vi "GeoData.vi"() -> ()   [LabVIEW 2017] (continued)
Pence springs\tWV\tSummers County\tH1\n24943\t54089\tGrassy meadows\tWV\tSummers County\tH1\n26330\t54091\tBridgeport\tWV\tTaylor County\tH1\n26374\t54091\tIndependence\tWV\tTaylor County\tH1\n26416\t54091\tPhilippi\tWV\tTaylor County\tH1\n26435\t54091\tSimpson\tWV\tTaylor County\tH1\n26354\t54091\tGrafton\tWV\tTaylor County\tH1\n26347\t54091\tFlemington\tWV\tTaylor County\tH1\n26554\t54091\tFairmont\tWV\tTaylor County\tH1\n26440\t54091\tThornton\tWV\tTaylor County\tH1\n26431\t54091\tShinnston\tWV\tTaylor County\tH1\n26424\t54091\tRosemont\tWV\tTaylor County\tH1\n26287\t54093\tParsons\tWV\tTucker County\tH1\n26271\t54093\tHendricks\tWV\tTucker County\tH1\n26263\t54093\tDryfork\tWV\tTucker County\tH1\n26254\t54093\tBowden\tWV\tTucker County\tH1\n26260\t54093\tDavis\tWV\tTucker County\tH1\n26289\t54093\tRed creek\tWV\tTucker County\tH1\n26283\t54093\tMontrose\tWV\tTucker County\tH1\n26276\t54093\tKerens\tWV\tTucker County\tH1\n26269\t54093\tHambleton\tWV\tTucker County\tH1\n26270\t54093\tHarman\tWV\tTucker County\tH1\n26292\t54093\tThomas\tWV\tTucker County\tH1\n26170\t54095\tSaint marys\tWV\tTyler County\tH1\n26415\t54095\tPennsboro\tWV\tTyler County\tH1\n26456\t54095\tWest union\tWV\tTyler County\tH1\n26155\t54095\tNew martinsville\tWV\tTyler County\tH1\n26159\t54095\tPaden city\tWV\tTyler County\tH1\n26175\t54095\tSistersville\tWV\tTyler County\tH1\n26149\t54095\tMiddlebourne\tWV\tTyler County\tH1\n26320\t54095\tAlma\tWV\tTyler County\tH1\n26167\t54095\tReader\tWV\tTyler County\tH1\n26377\t54095\tJacksonburg\tWV\tTyler County\tH1\n26146\t54095\tFriendly\tWV\tTyler County\tH1\n26434\t54095\tShirley\tWV\tTyler County\tH1\n26267\t54097\tEllamore\tWV\tUpshur County\tH1\n26218\t54097\tFrench creek\tWV\tUpshur County\tH1\n26385\t54097\tLost creek\tWV\tUpshur County\tH1\n26372\t54097\tHorner\tWV\tUpshur County\tH1\n26215\t54097\tCleveland\tWV\tUpshur County\tH1\n26236\t54097\tSelbyville\tWV\tUpshur County\tH1\n26210\t54097\tAdrian\tWV\tUpshur County\tH1\n26201\t54097\tBuckhannon\tWV\tUpshur County\tH1\n26343\t54097\tCrawford\tWV\tUpshur County\tH1\n26228\t54097\tKanawha head\tWV\tUpshur County\tH1\n26229\t54097\tLorentz\tWV\tUpshur County\tH1\n26234\t54097\tRock cave\tWV\tUpshur County\tH1\n26238\t54097\tVolga\tWV\tUpshur County\tH1\n26237\t54097\tTallmansville\tWV\tUpshur County\tH1\n25504\t54099\tBarboursville\tWV\tWayne County\tH1\n25530\t54099\tKenova\tWV\tWayne County\tH1\n25701\t54099\tHuntington\tWV\tWayne County\tH1\n25704\t54099\tHuntington\tWV\tWayne County\tH1\n25514\t54099\tFort gay\tWV\tWayne County\tH1\n25517\t54099\tGenoa\tWV\tWayne County\tH1\n25555\t54099\tPrichard\tWV\tWayne County\tH1\n25699\t54099\tWilsondale\tWV\tWayne County\tH1\n25524\t54099\tHarts\tWV\tWayne County\tH1\n25511\t54099\tDunlow\tWV\tWayne County\tH1\n25669\t54099\tCrum\tWV\tWayne County\tH1\n25562\t54099\tShoals\tWV\tWayne County\tH1\n25671\t54099\tDingess\tWV\tWayne County\tH1\n25534\t54099\tKiahsville\tWV\tWayne County\tH1\n25512\t54099\tEast lynn\tWV\tWayne County\tH1\n25570\t54099\tWayne\tWV\tWayne County\tH1\n25535\t54099\tLavalette\tWV\tWayne County\tH1\n25557\t54099\tRanger\tWV\tWayne County\tH1\n25507\t54099\tCeredo\tWV\tWayne County\tH1\n25674\t54099\tKermit\tWV\tWayne County\tH1\n25506\t54099\tBranchland\tWV\tWayne County\tH1\n26217\t54101\tDiana\tWV\tWebster County\tH1\n26203\t54101\tErbacon\tWV\tWebster County\tH1\n26266\t54101\tUpperglade\tWV\tWebster County\tH1\n26288\t54101\tWebster springs\tWV\tWebster County\tH1\n26208\t54101\tCamden on gauley\tWV\tWebster County\tH1\n26610\t54101\tBirch river\tWV\tWebster County\tH1\n26222\t54101\tHacker valley\tWV\tWebster County\tH1\n26206\t54101\tCowen\tWV\tWebster County\tH1\n26298\t54101\tBergoo\tWV\tWebster County\tH1\n26033\t54103\tCameron\tWV\tWetzel County\tH1\n26562\t54103\tBurton\tWV\tWetzel County\tH1\n26582\t54103\tMannington\tWV\tWetzel County\tH1\n26581\t54103\tLittleton\tWV\tWetzel County\tH1\n26437\t54103\tSmithfield\tWV\tWetzel County\tH1\n26162\t54103\tPorters falls\tWV\tWetzel County\tH1\n26155\t54103\tNew martinsville\tWV\tWetzel County\tH1\n26585\t54103\tMetz\tWV\tWetzel County\tH1\n26159\t54103\tPaden city\tWV\tWetzel County\tH1\n26575\t54103\tHundred\tWV\tWetzel County\tH1\n26561\t54103\tBig run\tWV\tWetzel County\tH1\n26055\t54103\tProctor\tWV\tWetzel County\tH1\n26149\t54103\tMiddlebourne\tWV\tWetzel County\tH1\n26348\t54103\tFolsom\tWV\tWetzel County\tH1\n26167\t54103\tReader\tWV\tWetzel County\tH1\n26377\t54103\tJacksonburg\tWV\tWetzel County\tH1\n26419\t54103\tPine grove\tWV\tWetzel County\tH1\n25252\t54105\tLe roy\tWV\tWirt County\tH1\n26180\t54105\tWalker\tWV\tWirt County\tH1\n25275\t54105\tSandyville\tWV\tWirt County\tH1\n26161\t54105\tPetroleum\tWV\tWirt County\tH1\n26141\t54105\tCreston\tWV\tWirt County\tH1\n26143\t54105\tElizabeth\tWV\tWirt County\tH1\n26160\t54105\tPalestine\tWV\tWirt County\tH1\n26152\t54105\tMunday\tWV\tWirt County\tH1\n25270\t54105\tReedy\tWV\tWirt County\tH1\n26138\t54105\tBrohard\tWV\tWirt County\tH1\n26169\t54107\tRockport\tWV\tWood County\tH1\n26170\t54107\tSaint marys\tWV\tWood County\tH1\n26184\t54107\tWaverly\tWV\tWood County\tH1\n26180\t54107\tWalker\tWV\tWood County\tH1\n26102\t54107\tParkersburg\tWV\tWood County\tH1\n26101\t54107\tParkersburg\tWV\tWood County\tH1\n26164\t54107\tRavenswood\tWV\tWood County\tH1\n26142\t54107\tDavisville\tWV\tWood County\tH1\n26103\t54107\tParkersburg\tWV\tWood County\tH1\n26150\t54107\tMineral wells\tWV\tWood County\tH1\n26120\t54107\tMineral wells\tWV\tWood County\tH1\n26104\t54107\tParkersburg\tWV\tWood County\tH1\n26181\t54107\tWashington\tWV\tWood County\tH1\n26143\t54107\tElizabeth\tWV\tWood County\tH1\n26187\t54107\tWilliamstown\tWV\tWood County\tH1\n26106\t54107\tParkersburg\tWV\tWood County\tH1\n26133\t54107\tBelleville\tWV\tWood County\tH1\n26121\t54107\tMineral wells\tWV\tWood County\tH1\n26105\t54107\tVienna\tWV\tWood County\tH1\n24870\t54109\tOceana\tWV\tWyoming County\tH1\n25882\t54109\tMullens\tWV\tWyoming County\tH1\n25617\t54109\tDavin\tWV\tWyoming County\tH1\n24716\t54109\tBud\tWV\tWyoming County\tH1\n25875\t54109\tMc graws\tWV\tWyoming County\tH1\n24726\t54109\tHerndon\tWV\tWyoming County\tH1\n24827\t54109\tCyclone\tWV\tWyoming County\tH1\n25870\t54109\tMaben\tWV\tWyoming County\tH1\n24898\t54109\tWyoming\tWV\tWyoming County\tH1\n25943\t54109\tWyco\tWV\tWyoming County\tH1\n24828\t54109\tDavy\tWV\tWyoming County\tH1\n25928\t54109\tStephenson\tWV\tWyoming County\tH1\n25826\t54109\tCorinne\tWV\tWyoming County\tH1\n25810\t54109\tAllen junction\tWV\tWyoming County\tH1\n24857\t54109\tLynco\tWV\tWyoming County\tH1\n25876\t54109\tSaulsville\tWV\tWyoming County\tH1\n24882\t54109\tSimon\tWV\tWyoming County\tH1\n25913\t54109\tRavencliff\tWV\tWyoming County\tH1\n24854\t54109\tKopperston\tWV\tWyoming County\tH1\n24736\t54109\tMatoaka\tWV\tWyoming County\tH1\n24839\t54109\tHanover\tWV\tWyoming County\tH1\n24849\t54109\tJesse\tWV\tWyoming County\tH1\n25848\t54109\tGlen rogers\tWV\tWyoming County\tH1\n24818\t54109\tBrenton\tWV\tWyoming County\tH1\n24822\t54109\tClear fork\tWV\tWyoming County\tH1\n24869\t54109\tNorth spring\tWV\tWyoming County\tH1\n24880\t54109\tRock view\tWV\tWyoming County\tH1\n25845\t54109\tGlen fork\tWV\tWyoming County\tH1\n24845\t54109\tIkes fork\tWV\tWyoming County\tH1\n24801\t54109\tWelch\tWV\tWyoming County\tH1\n24872\t54109\tPanther\tWV\tWyoming County\tH1\n24823\t54109\tCoal mountain\tWV\tWyoming County\tH1\n24860\t54109\tMatheny\tWV\tWyoming County\tH1\n24719\t54109\tCovel\tWV\tWyoming County\tH1\n25811\t54109\tAmigo\tWV\tWyoming County\tH1\n24844\t54109\tIaeger\tWV\tWyoming County\tH1\n24874\t54109\tPineville\tWV\tWyoming County\tH1\n25916\t54109\tSabine\tWV\tWyoming County\tH1\n24867\t54109\tNew richmond\tWV\tWyoming County\tH1\n24847\t54109\tItmann\tWV\tWyoming County\tH1\n24834\t54109\tFanrock\tWV\tWyoming County\tH1\n53936\t55001\tGrand marsh\tWI\tAdams County\tH1\n53934\t55001\tFriendship\tWI\tAdams County\tH1\n54613\t55001\tArkdale\tWI\tAdams County\tH1\n53910\t55001\tAdams\tWI\tAdams County\tH1\n54930\t55001\tColoma\tWI\tAdams County\tH1\n53920\t55001\tBriggsville\tWI\tAdams County\tH1\n54966\t55001\tPlainfield\tWI\tAdams County\tH1\n54943\t55001\tHancock\tWI\tAdams County\tH1\n53965\t55001\tWisconsin dells\tWI\tAdams County\tH1\n53952\t55001\tOxford\tWI\tAdams County\tH1\n54921\t55001\tBancroft\tWI\tAdams County\tH1\n54457\t55001\tNekoosa\tWI\tAdams County\tH1\n54494\t55001\tWisconsin rapids\tWI\tAdams County\tH1\n53964\t55001\tWestfield\tWI\tAdams County\tH1\n54646\t55001\tNecedah\tWI\tAdams County\tH1\n54559\t55003\tSaxon\tWI\tAshland County\tH1\n54806\t55003\tAshland\tWI\tAshland County\tH1\n54855\t55003\tMarengo\tWI\tAshland County\tH1\n54846\t55003\tHigh bridge\tWI\tAshland County\tH1\n54850\t55003\tLa pointe\tWI\tAshland County\tH1\n54517\t55003\tClam lake\tWI\tAshland County\tH1\n54527\t55003\tGlidden\tWI\tAshland County\tH1\n54514\t55003\tButternut\tWI\tAshland County\tH1\n54546\t55003\tMellen\tWI\tAshland County\tH1\n54856\t55003\tMason\tWI\tAshland County\tH1\n54861\t55003\tOdanah\tWI\tAshland County\tH1\n54004\t55005\tClayton\tWI\tBarron County\tH1\n54826\t55005\tComstock\tWI\tBarron County\tH1\n54889\t55005\tTurtle lake\tWI\tBarron County\tH1\n54813\t55005\tBarronett\tWI\tBarron County\tH1\n54841\t55005\tHaugen\tWI\tBarron County\tH1\n54728\t55005\tChetek\tWI\tBarron County\tH1\n54757\t55005\tNew auburn\tWI\tBarron County\tH1\n54733\t55005\tDallas\tWI\tBarron County\tH1\n54868\t55005\tRice lake\tWI\tBarron County\tH1\n54805\t55005\tAlmena\tWI\tBarron County\tH1\n54763\t55005\tRidgeland\tWI\tBarron County\tH1\n54812\t55005\tBarron\tWI\tBarron County\tH1\n54005\t55005\tClear lake\tWI\tBarron County\tH1\n54870\t55005\tSarona\tWI\tBarron County\tH1\n54857\t55005\tMikana\tWI\tBarron County\tH1\n54822\t55005\tCameron\tWI\tBarron County\tH1\n54762\t55005\tPrairie farm\tWI\tBarron County\tH1\n54829\t55005\tCumberland\tWI\tBarron County\tH1\n54817\t55005\tBirchwood\tWI\tBarron County\tH1\n54891\t55007\tWashburn\tWI\tBayfield County\tH1\n54844\t55007\tHerbster\tWI\tBayfield County\tH1\n54847\t55007\tIron river\tWI\tBayfield County\tH1\n54806\t55007\tAshland\tWI\tBayfield County\tH1\n54839\t55007\tGrand view\tWI\tBayfield County\tH1\n54821\t55007\tCable\tWI\tBayfield County\tH1\n54827\t55007\tCornucopia\tWI\tBayfield County\tH1\n54814\t55007\tBayfield\tWI\tBayfield County\tH1\n54820\t55007\tBrule\tWI\tBayfield County\tH1\n54873\t55007\tSolon springs\tWI\tBayfield County\tH1\n54832\t55007\tDrummond\tWI\tBayfield County\tH1\n54838\t55007\tGordon\tWI\tBayfield County\tH1\n54816\t55007\tBenoit\tWI\tBayfield County\tH1\n54856\t55007\tMason\tWI\tBayfield County\tH1\n54865\t55007\tPort wing\tWI\tBayfield County\tH1\n54324\t55009\tGreen bay\tWI\tBrown County\tH1\n54307\t55009\tGreen bay\tWI\tBrown County\tH1\n54130\t55009\tKaukauna\tWI\tBrown County\tH1\n54155\t55009\tOneida\tWI\tBrown County\tH1\n54126\t55009\tGreenleaf\tWI\tBrown County\tH1\n54304\t55009\tGreen bay\tWI\tBrown County\tH1\n54302\t55009\tGreen bay\tWI\tBrown County\tH1\n54180\t55009\tWrightstown\tWI\tBrown County\tH1\n54110\t55009\tBrillion\tWI\tBrown County\tH1\n54229\t55009\tNew franken\tWI\tBrown County\tH1\n54301\t55009\tGreen bay\tWI\tBrown County\tH1\n54311\t55009\tGreen bay\tWI\tBrown County\tH1\n54305\t55009\tGreen bay\tWI\tBrown County\tH1\n54115\t55009\tDe pere\tWI\tBrown County\tH1\n54173\t55009\tSuamico\tWI\tBrown County\tH1\n54230\t55009\tReedsville\tWI\tBrown County\tH1\n54313\t55009\tGreen bay\tWI\tBrown County\tH1\n54227\t55009\tMaribel\tWI\tBrown County\tH1\n54217\t55009\tLuxemburg\tWI\tBrown County\tH1\n54208\t55009\tDenmark\tWI\tBrown County\tH1\n54165\t55009\tSeymour\tWI\tBrown County\tH1\n54303\t55009\tGreen bay\tWI\tBrown County\tH1\n54162\t55009\tPulaski\tWI\tBrown County\tH1\n54308\t55009\tGreen bay\tWI\tBrown County\tH1\n54344\t55009\tGreen bay\tWI\tBrown County\tH1\n54622\t55011\tCochrane\tWI\tBuffalo County\tH1\n54612\t55011\tArcadia\tWI\tBuffalo County\tH1\n54738\t55011\tEleva\tWI\tBuffalo County\tH1\n54747\t55011\tIndependence\tWI\tBuffalo County\tH1\n54743\t55011\tGilmanton\tWI\tBuffalo County\tH1\n54736\t55011\tDurand\tWI\tBuffalo County\tH1\n54756\t55011\tNelson\tWI\tBuffalo County\tH1\n54629\t55011\tFountain city\tWI\tBuffalo County\tH1\n54610\t55011\tAlma\tWI\tBuffalo County\tH1\n54755\t55011\tMondovi\tWI\tBuffalo County\tH1\n54830\t55013\tDanbury\tWI\tBurnett County\tH1\n54813\t55013\tBarronett\tWI\tBurnett County\tH1\n54837\t55013\tFrederic\tWI\tBurnett County\tH1\n54871\t55013\tShell lake\tWI\tBurnett County\tH1\n54840\t55013\tGrantsburg\tWI\tBurnett County\tH1\n54893\t55013\tWebster\tWI\tBurnett County\tH1\n54888\t55013\tTrego\tWI\tBurnett County\tH1\n54024\t55013\tSaint croix falls\tWI\tBurnett County\tH1\n54872\t55013\tSiren\tWI\tBurnett County\tH1\n54801\t55013\tSpooner\tWI\tBurnett County\tH1\n54859\t55013\tMinong\tWI\tBurnett County\tH1\n54845\t55013\tHertel\tWI\tBurnett County\tH1\n54853\t55013\tLuck\tWI\tBurnett County\tH1\n53088\t55015\tStockbridge\tWI\tCalumet County\tH1\n54130\t55015\tKaukauna\tWI\tCalumet County\tH1\n53062\t55015\tNew holstein\tWI\tCalumet County\tH1\n54110\t55015\tBrillion\tWI\tCalumet County\tH1\n53014\t55015\tChilton\tWI\tCalumet County\tH1\n53042\t55015\tKiel\tWI\tCalumet County\tH1\n54160\t55015\tPotter\tWI\tCalumet County\tH1\n53079\t55015\tSaint cloud\tWI\tCalumet County\tH1\n54169\t55015\tSherwood\tWI\tCalumet County\tH1\n54123\t55015\tForest junction\tWI\tCalumet County\tH1\n53020\t55015\tElkhart lake\tWI\tCalumet County\tH1\n54915\t55015\tAppleton\tWI\tCalumet County\tH1\n53061\t55015\tNew holstein\tWI\tCalumet County\tH1\n53049\t55015\tMalone\tWI\tCalumet County\tH1\n54129\t55015\tHilbert\tWI\tCalumet County\tH1\n54952\t55015\tMenasha\tWI\tCalumet County\tH1\n54748\t55017\tJim falls\tWI\tChippewa County\tH1\n54727\t55017\tCadott\tWI\tChippewa County\tH1\n54729\t55017\tChippewa falls\tWI\tChippewa County\tH1\n54732\t55017\tCornell\tWI\tChippewa County\tH1\n54745\t55017\tHolcombe\tWI\tChippewa County\tH1\n54757\t55017\tNew auburn\tWI\tChippewa County\tH1\n54739\t55017\tElk mound\tWI\tChippewa County\tH1\n54703\t55017\tEau claire\tWI\tChippewa County\tH1\n54724\t55017\tBloomer\tWI\tChippewa County\tH1\n54730\t55017\tColfax\tWI\tChippewa County\tH1\n54433\t55017\tGilman\tWI\tChippewa County\tH1\n54726\t55017\tBoyd\tWI\tChippewa County\tH1\n54768\t55017\tStanley\tWI\tChippewa County\tH1\n54766\t55017\tSheldon\tWI\tChippewa County\tH1\n54774\t55017\tChippewa falls\tWI\tChippewa County\tH1\n54446\t55019\tLoyal\tWI\tClark County\tH1\n54741\t55019\tFairchild\tWI\tClark County\tH1\n54420\t55019\tChili\tWI\tClark County\tH1\n54771\t55019\tThorp\tWI\tClark County\tH1\n54436\t55019\tGranton\tWI\tClark County\tH1\n54425\t55019\tDorchester\tWI\tClark County\tH1\n54498\t55019\tWithee\tWI\tClark County\tH1\n54754\t55019\tMerrillan\tWI\tClark County\tH1\n54746\t55019\tHumbird\tWI\tClark County\tH1\n54460\t55019\tOwen\tWI\tClark County\tH1\n54479\t55019\tSpencer\tWI\tClark County\tH1\n54456\t55019\tNeillsville\tWI\tClark County\tH1\n54488\t55019\tUnity\tWI\tClark County\tH1\n54449\t55019\tMarshfield\tWI\tClark County\tH1\n54421\t55019\tColby\tWI\tClark County\tH1\n54493\t55019\tWillard\tWI\tClark County\tH1\n54768\t55019\tStanley\tWI\tClark County\tH1\n54422\t55019\tCurtiss\tWI\tClark County\tH1\n54437\t55019\tGreenwood\tWI\tClark County\tH1\n54466\t55019\tPittsville\tWI\tClark County\tH1\n54405\t55019\tAbbotsford\tWI\tClark County\tH1\n53932\t55021\tFall river\tWI\tColumbia County\tH1\n53935\t55021\tFriesland\tWI\tColumbia County\tH1\n53561\t55021\tMerrimac\tWI\tColumbia County\tH1\n53954\t55021\tPardeeville\tWI\tColumbia County\tH1\n53911\t55021\tArlington\tWI\tColumbia County\tH1\n53969\t55021\tWyocena\tWI\tColumbia County\tH1\n53901\t55021\tPortage\tWI\tColumbia County\tH1\n53956\t55021\tRandolph\tWI\tColumbia County\tH1\n53960\t55021\tRio\tWI\tColumbia County\tH1\n53555\t55021\tLodi\tWI\tColumbia County\tH1\n53955\t55021\tPoynette\tWI\tColumbia County\tH1\n53925\t55021\tColumbus\tWI\tColumbia County\tH1\n53965\t55021\tWisconsin dells\tWI\tColumbia County\tH1\n53926\t55021\tDalton\tWI\tColumbia County\tH1\n53957\t55021\tRandolph\tWI\tColumbia County\tH1\n53583\t55021\tSauk city\tWI\tColumbia County\tH1\n53578\t55021\tPrairie du sac\tWI\tColumbia County\tH1\n53913\t55021\tBaraboo\tWI\tColumbia County\tH1\n53923\t55021\tCambria\tWI\tColumbia County\tH1\n53571\t55021\tMorrisonville\tWI\tColumbia County\tH1\n53928\t55021\tDoylestown\tWI\tColumbia County\tH1\n53532\t55021\tDeforest\tWI\tColumbia County\tH1\n54657\t55023\tSteuben\tWI\tCrawford County\tH1\n53821\t55023\tPrairie du chien\tWI\tCrawford County\tH1\n54631\t55023\tGays mills\tWI\tCrawford County\tH1\n54655\t55023\tSoldiers grove\tWI\tCrawford County\tH1\n53518\t55023\tBlue river\tWI\tCrawford County\tH1\n54624\t55023\tDe soto\tWI\tCrawford County\tH1\n54665\t55023\tViroqua\tWI\tCrawford County\tH1\n54654\t55023\tSeneca\tWI\tCrawford County\tH1\n53805\t55023\tBoscobel\tWI\tCrawford County\tH1\n54626\t55023\tEastman\tWI\tCrawford County\tH1\n54652\t55023\tReadstown\tWI\tCrawford County\tH1\n54645\t55023\tMount sterling\tWI\tCrawford County\tH1\n53826\t55023\tWauzeka\tWI\tCrawford County\tH1\n54628\t55023\tFerryville\tWI\tCrawford County\tH1\n53521\t55025\tBrooklyn\tWI\tDane County\tH1\n53517\t55025\tBlue mounds\tWI\tDane County\tH1\n53715\t55025\tMadison\tWI\tDane County\tH1\n53716\t55025\tMadison\tWI\tDane County\tH1\n53718\t55025\tMadison\tWI\tDane County\tH1\n53594\t55025\tWaterloo\tWI\tDane County\tH1\n53516\t55025\tBlanchardville\tWI\tDane County\tH1\n53704\t55025\tMadison\tWI\tDane County\tH1\n53713\t55025\tMadison\tWI\tDane County\tH1\n53714\t55025\tMadison\tWI\tDane County\tH1\n53572\t55025\tMount horeb\tWI\tDane County\tH1\n53558\t55025\tMc farland\tWI\tDane County\tH1\n53575\t55025\tOregon\tWI\tDane County\tH1\n53744\t55025\tMadison\tWI\tDane County\tH1\n53792\t55025\tMadison\tWI\tDane County\tH1\n53703\t55025\tMadison\tWI\tDane County\tH1\n53590\t55025\tSun prairie\tWI\tDane County\tH1\n53597\t55025\tWaunakee\tWI\tDane County\tH1\n53593\t55025\tVerona\tWI\tDane County\tH1\n53911\t55025\tArlington\tWI\tDane County\tH1\n53701\t55025\tMadison\tWI\tDane County\tH1\n53777\t55025\tMadison\tWI\tDane County\tH1\n53783\t55025\tMadison\tWI\tDane County\tH1\n53508\t55025\tBelleville\tWI\tDane County\tH1\n53705\t55025\tMadison\tWI\tDane County\tH1\n53562\t55025\tMiddleton\tWI\tDane County\tH1\n53559\t55025\tMarshall\tWI\tDane County\tH1\n53560\t55025\tMazomanie\tWI\tDane County\tH1\n53596\t55025\tSun prairie\tWI\tDane County\tH1\n53788\t55025\tMadison\tWI\tDane County\tH1\n53527\t55025\tCottage grove\tWI\tDane County\tH1\n53528\t55025\tCross plains\tWI\tDane County\tH1\n53515\t55025\tBlack earth\tWI\tDane County\tH1\n53719\t55025\tMadison\tWI\tDane County\tH1\n53960\t55025\tRio\tWI\tDane County\tH1\n53707\t55025\tMadison\tWI\tDane County\tH1\n53523\t55025\tCambridge\tWI\tDane County\tH1\n53529\t55025\tDane\tWI\tDane County\tH1\n53589\t55025\tStoughton\tWI\tDane County\tH1\n53708\t55025\tMadison\tWI\tDane County\tH1\n53555\t55025\tLodi\tWI\tDane County\tH1\n53574\t55025\tNew glarus\tWI\tDane County\tH1\n53726\t55025\tMadison\tWI\tDane County\tH1\n53925\t55025\tColumbus\tWI\tDane County\tH1\n53725\t55025\tMadison\tWI\tDane County\tH1\n53784\t55025\tMadison\tWI\tDane County\tH1\n53583\t55025\tSauk city\tWI\tDane County\tH1\n53717\t55025\tMadison\tWI\tDane County\tH1\n53598\t55025\tWindsor\tWI\tDane County\tH1\n53706\t55025\tMadison\tWI\tDane County\tH1\n53571\t55025\tMorrisonville\tWI\tDane County\tH1\n53507\t55025\tBarneveld\tWI\tDane County\tH1\n53544\t55025\tHollandale\tWI\tDane County\tH1\n53534\t55025\tEdgerton\tWI\tDane County\tH1\n53531\t55025\tDeerfield\tWI\tDane County\tH1\n53532\t55025\tDeforest\tWI\tDane County\tH1\n53711\t55025\tMadison\tWI\tDane County\tH1\n53702\t55025\tMadison\tWI\tDane County\tH1\n53027\t55027\tHartford\tWI\tDodge County\tH1\n53034\t55027\tHustisford\tWI\tDodge County\tH1\n53594\t55027\tWaterloo\tWI\tDodge County\tH1\n53932\t55027\tFall river\tWI\tDodge County\tH1\n53579\t55027\tReeseville\tWI\tDodge County\tH1\n53557\t55027\tLowell\tWI\tDodge County\tH1\n53066\t55027\tOconomowoc\tWI\tDodge County\tH1\n53035\t55027\tIron ridge\tWI\tDodge County\tH1\n53963\t55027\tWaupun\tWI\tDodge County\tH1\n53010\t55027\tCampbellsport\tWI\tDodge County\tH1\n53099\t55027\tWoodland\tWI\tDodge County\tH1\n53078\t55027\tRubicon\tWI\tDodge County\tH1\n53933\t55027\tFox lake\tWI\tDodge County\tH1\n53006\t55027\tBrownsville\tWI\tDodge County\tH1\n53047\t55027\tLebanon\tWI\tDodge County\tH1\n53091\t55027\tTheresa\tWI\tDodge County\tH1\n53059\t55027\tNeosho\tWI\tDodge County\tH1\n53946\t55027\tMarkesan\tWI\tDodge County\tH1\n53003\t55027\tAshippun\tWI\tDodge County\tH1\n53094\t55027\tWatertown\tWI\tDodge County\tH1\n53048\t55027\tLomira\tWI\tDodge County\tH1\n53036\t55027\tIxonia\tWI\tDodge County\tH1\n53956\t55027\tRandolph\tWI\tDodge County\tH1\n53032\t55027\tHoricon\tWI\tDodge County\tH1\n53016\t55027\tClyman\tWI\tDodge County\tH1\n53039\t55027\tJuneau\tWI\tDodge County\tH1\n53098\t55027\tWatertown\tWI\tDodge County\tH1\n53925\t55027\tColumbus\tWI\tDodge County\tH1\n53922\t55027\tBurnett\tWI\tDodge County\tH1\n53050\t55027\tMayville\tWI\tDodge County\tH1\n53916\t55027\tBeaver dam\tWI\tDodge County\tH1\n53065\t55027\tOakfield\tWI\tDodge County\tH1\n54210\t55029\tEllison bay\tWI\tDoor County\tH1\n54202\t55029\tBaileys harbor\tWI\tDoor County\tH1\n54211\t55029\tEphraim\tWI\tDoor County\tH1\n54234\t55029\tSister bay\tWI\tDoor County\tH1\n54226\t55029\tMaplewood\tWI\tDoor County\tH1\n54205\t55029\tCasco\tWI\tDoor County\tH1\n54235\t55029\tSturgeon bay\tWI\tDoor County\tH1\n54209\t55029\tEgg harbor\tWI\tDoor County\tH1\n54213\t55029\tForestville\tWI\tDoor County\tH1\n54217\t55029\tLuxemburg\tWI\tDoor County\tH1\n54201\t55029\tAlgoma\tWI\tDoor County\tH1\n54204\t55029\tBrussels\tWI\tDoor County\tH1\n54212\t55029\tFish creek\tWI\tDoor County\tH1\n54246\t55029\tWashington island\tWI\tDoor County\tH1\n54849\t55031\tLake nebagamon\tWI\tDouglas County\tH1\n54890\t55031\tWascott\tWI\tDouglas County\tH1\n54880\t55031\tSuperior\tWI\tDouglas County\tH1\n54830\t55031\tDanbury\tWI\tDouglas County\tH1\n54854\t55031\tMaple\tWI\tDouglas County\tH1\n54874\t55031\tSouth range\tWI\tDouglas County\tH1\n54864\t55031\tPoplar\tWI\tDouglas County\tH1\n54842\t55031\tHawthorne\tWI\tDouglas County\tH1\n54820\t55031\tBrule\tWI\tDouglas County\tH1\n54873\t55031\tSolon springs\tWI\tDouglas County\tH1\n54838\t55031\tGordon\tWI\tDouglas County\tH1\n54859\t55031\tMinong\tWI\tDouglas County\tH1\n54836\t55031\tFoxboro\tWI\tDouglas County\tH1\n54721\t55033\tArkansaw\tWI\tDunn County\tH1\n54735\t55033\tDownsville\tWI\tDunn County\tH1\n54749\t55033\tKnapp\tWI\tDunn County\tH1\n54027\t55033\tWilson\tWI\tDunn County\tH1\n54751\t55033\tMenomonie\tWI\tDunn County\tH1\n54728\t55033\tChetek\tWI\tDunn County\tH1\n54757\t55033\tNew auburn\tWI\tDunn County\tH1\n54772\t55033\tWheeler\tWI\tDunn County\tH1\n54739\t55033\tElk mound\tWI\tDunn County\tH1\n54761\t55033\tPlum city\tWI\tDunn County\tH1\n54765\t55033\tSand creek\tWI\tDunn County\tH1\n54703\t55033\tEau claire\tWI\tDunn County\tH1\n54724\t55033\tBloomer\tWI\tDunn County\tH1\n54730\t55033\tColfax\tWI\tDunn County\tH1\n54725\t55033\tBoyceville\tWI\tDunn County\tH1\n54736\t55033\tDurand\tWI\tDunn County\tH1\n54763\t55033\tRidgeland\tWI\tDunn County\tH1\n54013\t55033\tGlenwood city\tWI\tDunn County\tH1\n54005\t55033\tClear lake\tWI\tDunn County\tH1\n54740\t55033\tElmwood\tWI\tDunn County\tH1\n54734\t55033\tDowning\tWI\tDunn County\tH1\n54767\t55033\tSpring valley\tWI\tDunn County\tH1\n54737\t55033\tEau galle\tWI\tDunn County\tH1\n54701\t55033\tEau claire\tWI\tDunn County\tH1\n54755\t55033\tMondovi\tWI\tDunn County\tH1\n54762\t55033\tPrairie farm\tWI\tDunn County\tH1\n54764\t55033\tRock falls\tWI\tDunn County\tH1\n54741\t55035\tFairchild\tWI\tEau Claire County\tH1\n54727\t55035\tCadott\tWI\tEau Claire County\tH1\n54722\t55035\tAugusta\tWI\tEau Claire County\tH1\n54729\t55035\tChippewa falls\tWI\tEau Claire County\tH1\n54770\t55035\tStrum\tWI\tEau Claire County\tH1\n54739\t55035\tElk mound\tWI\tEau Claire County\tH1\n54738\t55035\tEleva\tWI\tEau Claire County\tH1\n54703\t55035\tEau claire\tWI\tEau Claire County\tH1\n54742\t55035\tFall creek\tWI\tEau Claire County\tH1\n54758\t55035\tOsseo\tWI\tEau Claire County\tH1\n54702\t55035\tEau claire\tWI\tEau Claire County\tH1\n54726\t55035\tBoyd\tWI\tEau Claire County\tH1\n54768\t55035\tStanley\tWI\tEau Claire County\tH1\n54701\t55035\tEau claire\tWI\tEau Claire County\tH1\n54720\t55035\tAltoona\tWI\tEau Claire County\tH1\n54755\t55035\tMondovi\tWI\tEau Claire County\tH1\n54151\t55037\tNiagara\tWI\tFlorence County\tH1\n54542\t55037\tLong lake\tWI\tFlorence County\tH1\n54120\t55037\tFence\tWI\tFlorence County\tH1\n54121\t55037\tFlorence\tWI\tFlorence County\tH1\n54103\t55037\tArmstrong creek\tWI\tFlorence County\tH1\n54904\t55039\tOshkosh\tWI\tFond du Lac County\tH1\n53963\t55039\tWaupun\tWI\tFond du Lac County\tH1\n53010\t55039\tCampbellsport\tWI\tFond du Lac County\tH1\n54937\t55039\tFond du lac\tWI\tFond du Lac County\tH1\n53014\t55039\tChilton\tWI\tFond du Lac County\tH1\n53006\t55039\tBrownsville\tWI\tFond du Lac County\tH1\n54979\t55039\tVan dyne\tWI\tFond du Lac County\tH1\n53946\t55039\tMarkesan\tWI\tFond du Lac County\tH1\n53023\t55039\tGlenbeulah\tWI\tFond du Lac County\tH1\n54932\t55039\tEldorado\tWI\tFond du Lac County\tH1\n54964\t55039\tPickett\tWI\tFond du Lac County\tH1\n53079\t55039\tSaint cloud\tWI\tFond du Lac County\tH1\n53048\t55039\tLomira\tWI\tFond du Lac County\tH1\n53011\t55039\tCascade\tWI\tFond du Lac County\tH1\n54935\t55039\tFond du lac\tWI\tFond du Lac County\tH1\n54971\t55039\tRipon\tWI\tFond du Lac County\tH1\n54936\t55039\tFond du lac\tWI\tFond du Lac County\tH1\n53919\t55039\tBrandon\tWI\tFond du Lac County\tH1\n53931\t55039\tFairwater\tWI\tFond du Lac County\tH1\n53065\t55039\tOakfield\tWI\tFond du Lac County\tH1\n53061\t55039\tNew holstein\tWI\tFond du Lac County\tH1\n53040\t55039\tKewaskum\tWI\tFond du Lac County\tH1\n53049\t55039\tMalone\tWI\tFond du Lac County\tH1\n53057\t55039\tMount calvary\tWI\tFond du Lac County\tH1\n53019\t55039\tEden\tWI\tFond du Lac County\tH1\n54974\t55039\tRosendale\tWI\tFond du Lac County\tH1\n54465\t55041\tPickerel\tWI\tForest County\tH1\n54511\t55041\tArgonne\tWI\tForest County\tH1\n54521\t55041\tEagle river\tWI\tForest County\tH1\n54542\t55041\tLong lake\tWI\tForest County\tH1\n54562\t55041\tThree lakes\tWI\tForest County\tH1\n54103\t55041\tArmstrong creek\tWI\tForest County\tH1\n54520\t55041\tCrandon\tWI\tForest County\tH1\n54566\t55041\tWabeno\tWI\tForest County\tH1\n54104\t55041\tAthelstane\tWI\tForest County\tH1\n54541\t55041\tLaona\tWI\tForest County\tH1\n53813\t55043\tLancaster\tWI\tGrant County\tH1\n53820\t55043\tPotosi\tWI\tGrant County\tH1\n53807\t55043\tCuba city\tWI\tGrant County\tH1\n53810\t55043\tGlen haven\tWI\tGrant County\tH1\n53821\t55043\tPrairie du chien\tWI\tGrant County\tH1\n53825\t55043\tStitzer\tWI\tGrant County\tH1\n53554\t55043\tLivingston\tWI\tGrant County\tH1\n53573\t55043\tMuscoda\tWI\tGrant County\tH1\n53817\t55043\tPatch grove\tWI\tGrant County\tH1\n53809\t55043\tFennimore\tWI\tGrant County\tH1\n53818\t55043\tPlatteville\tWI\tGrant County\tH1\n53569\t55043\tMontfort\tWI\tGrant County\tH1\n53827\t55043\tWoodman\tWI\tGrant County\tH1\n53801\t55043\tBagley\tWI\tGrant County\tH1\n53812\t55043\tKieler\tWI\tGrant County\tH1\n53802\t55043\tBeetown\tWI\tGrant County\tH1\n53518\t55043\tBlue river\tWI\tGrant County\tH1\n53811\t55043\tHazel green\tWI\tGrant County\tH1\n53824\t55043\tSinsinawa\tWI\tGrant County\tH1\n53805\t55043\tBoscobel\tWI\tGrant County\tH1\n53808\t55043\tDickeyville\tWI\tGrant County\tH1\n53543\t55043\tHighland\tWI\tGrant County\tH1\n53816\t55043\tMount hope\tWI\tGrant County\tH1\n53804\t55043\tBloomington\tWI\tGrant County\tH1\n53806\t55043\tCassville\tWI\tGrant County\tH1\n53521\t55045\tBrooklyn\tWI\tGreen County\tH1\n53502\t55045\tAlbany\tWI\tGreen County\tH1\n53516\t55045\tBlanchardville\tWI\tGreen County\tH1\n53522\t55045\tBrowntown\tWI\tGreen County\tH1\n53572\t55045\tMount horeb\tWI\tGreen County\tH1\n53520\t55045\tBrodhead\tWI\tGreen County\tH1\n53536\t55045\tEvansville\tWI\tGreen County\tH1\n53508\t55045\tBelleville\tWI\tGreen County\tH1\n53566\t55045\tMonroe\tWI\tGreen County\tH1\n53570\t55045\tMonticello\tWI\tGreen County\tH1\n53574\t55045\tNew glarus\tWI\tGreen County\tH1\n53504\t55045\tArgyle\tWI\tGreen County\tH1\n53544\t55045\tHollandale\tWI\tGreen County\tH1\n53550\t55045\tJuda\tWI\tGreen County\tH1\n53949\t55047\tMontello\tWI\tGreen Lake County\tH1\n54941\t55047\tGreen lake\tWI\tGreen Lake County\tH1\n53946\t55047\tMarkesan\tWI\tGreen Lake County\tH1\n54923\t55047\tBerlin\tWI\tGreen Lake County\tH1\n53956\t55047\tRandolph\tWI\tGreen Lake County\tH1\n53947\t55047\tMarquette\tWI\tGreen Lake County\tH1\n54971\t55047\tRipon\tWI\tGreen Lake County\tH1\n53919\t55047\tBrandon\tWI\tGreen Lake County\tH1\n53926\t55047\tDalton\tWI\tGreen Lake County\tH1\n53923\t55047\tCambria\tWI\tGreen Lake County\tH1\n54960\t55047\tNeshkoro\tWI\tGreen Lake County\tH1\n54968\t55047\tPrinceton\tWI\tGreen Lake County\tH1\n53939\t55047\tKingston\tWI\tGreen Lake County\tH1\n53517\t55049\tBlue mounds\tWI\tIowa County\tH1\n53506\t55049\tAvoca\tWI\tIowa County\tH1\n53516\t55049\tBlanchardville\tWI\tIowa County\tH1\n53572\t55049\tMount horeb\tWI\tIowa County\tH1\n53595\t55049\tDodgeville\tWI\tIowa County\tH1\n53553\t55049\tLinden\tWI\tIowa County\tH1\n53554\t55049\tLivingston\tWI\tIowa County\tH1\n53573\t55049\tMuscoda\tWI\tIowa County\tH1\n53565\t55049\tMineral point\tWI\tIowa County\tH1\n53560\t55049\tMazomanie\tWI\tIowa County\tH1\n53535\t55049\tEdmund\tWI\tIowa County\tH1\n53515\t55049\tBlack earth\tWI\tIowa County\tH1\n53818\t55049\tPlatteville\tWI\tIowa County\tH1\n53582\t55049\tRidgeway\tWI\tIowa County\tH1\n53569\t55049\tMontfort\tWI\tIowa County\tH1\n53580\t55049\tRewey\tWI\tIowa County\tH1\n53533\t55049\tDodgeville\tWI\tIowa County\tH1\n53588\t55049\tSpring green\tWI\tIowa County\tH1\n53507\t55049\tBarneveld\tWI\tIowa County\tH1\n53526\t55049\tCobb\tWI\tIowa County\tH1\n53503\t55049\tArena\tWI\tIowa County\tH1\n53543\t55049\tHighland\tWI\tIowa County\tH1\n53544\t55049\tHollandale\tWI\tIowa County\tH1\n54538\t55051\tLac du flambeau\tWI\tIron County\tH1\n54559\t55051\tSaxon\tWI\tIron County\tH1\n54534\t55051\tHurley\tWI\tIron County\tH1\n54525\t55051\tGile\tWI\tIron County\tH1\n54550\t55051\tMontreal\tWI\tIron County\tH1\n54536\t55051\tIron belt\tWI\tIron County\tH1\n54565\t55051\tUpson\tWI\tIron County\tH1\n54514\t55051\tButternut\tWI\tIron County\tH1\n54552\t55051\tPark falls\tWI\tIron County\tH1\n54547\t55051\tMercer\tWI\tIron County\tH1\n54741\t55053\tFairchild\tWI\tJackson County\tH1\n54666\t55053\tWarrens\tWI\tJackson County\tH1\n54643\t55053\tMillston\tWI\tJackson County\tH1\n54635\t55053\tHixton\tWI\tJackson County\tH1\n54754\t55053\tMerrillan\tWI\tJackson County\tH1\n54746\t55053\tHumbird\tWI\tJackson County\tH1\n54611\t55053\tAlma center\tWI\tJackson County\tH1\n54642\t55053\tMelrose\tWI\tJackson County\tH1\n54659\t55053\tTaylor\tWI\tJackson County\tH1\n54644\t55053\tMindoro\tWI\tJackson County\tH1\n54615\t55053\tBlack river falls\tWI\tJackson County\tH1\n54616\t55053\tBlair\tWI\tJackson County\tH1\n54758\t55053\tOsseo\tWI\tJackson County\tH1\n54627\t55053\tEttrick\tWI\tJackson County\tH1\n54466\t55053\tPittsville\tWI\tJackson County\tH1\n53563\t55055\tMilton\tWI\tJefferson County\tH1\n53549\t55055\tJefferson\tWI\tJefferson County\tH1\n53551\t55055\tLake mills\tWI\tJefferson County\tH1\n53594\t55055\tWaterloo\tWI\tJefferson County\tH1\n53066\t55055\tOconomowoc\tWI\tJefferson County\tH1\n53190\t55055\tWhitewater\tWI\tJefferson County\tH1\n53118\t55055\tDousman\tWI\tJefferson County\tH1\n53559\t55055\tMarshall\tWI\tJefferson County\tH1\n53094\t55055\tWatertown\tWI\tJefferson County\tH1\n53036\t55055\tIxonia\tWI\tJefferson County\tH1\n53098\t55055\tWatertown\tWI\tJefferson County\tH1\n53038\t55055\tJohnson creek\tWI\tJefferson County\tH1\n53523\t55055\tCambridge\tWI\tJefferson County\tH1\n53178\t55055\tSullivan\tWI\tJefferson County\tH1\n53156\t55055\tPalmyra\tWI\tJefferson County\tH1\n53119\t55055\tEagle\tWI\tJefferson County\tH1\n53538\t55055\tFort atkinson\tWI\tJefferson County\tH1\n53534\t55055\tEdgerton\tWI\tJefferson County\tH1\n53137\t55055\tHelenville\tWI\tJefferson County\tH1\n53968\t55057\tWonewoc\tWI\tJuneau County\tH1\n53950\t55057\tNew lisbon\tWI\tJuneau County\tH1\n54634\t55057\tHillsboro\tWI\tJuneau County\tH1\n54618\t55057\tCamp douglas\tWI\tJuneau County\tH1\n54666\t55057\tWarrens\tWI\tJuneau County\tH1\n54641\t55057\tMather\tWI\tJuneau County\tH1\n53929\t55057\tElroy\tWI\tJuneau County\tH1\n54637\t55057\tHustler\tWI\tJuneau County\tH1\n53944\t55057\tLyndon station\tWI\tJuneau County\tH1\n53965\t55057\tWisconsin dells\tWI\tJuneau County\tH1\n53948\t55057\tMauston\tWI\tJuneau County\tH1\n54457\t55057\tNekoosa\tWI\tJuneau County\tH1\n54638\t55057\tKendall\tWI\tJuneau County\tH1\n53962\t55057\tUnion center\tWI\tJuneau County\tH1\n53941\t55057\tLa valle\tWI\tJuneau County\tH1\n54646\t55057\tNecedah\tWI\tJuneau County\tH1\n53128\t55059\tGenoa city\tWI\tKenosha County\tH1\n53144\t55059\tKenosha\tWI\tKenosha County\tH1\n53140\t55059\tKenosha\tWI\tKenosha County\tH1\n53109\t55059\tCamp lake\tWI\tKenosha County\tH1\n53159\t55059\tPowers lake\tWI\tKenosha County\tH1\n53105\t55059\tBurlington\tWI\tKenosha County\tH1\n53403\t55059\tRacine\tWI\tKenosha County\tH1\n53182\t55059\tUnion grove\tWI\tKenosha County\tH1\n53168\t55059\tSalem\tWI\tKenosha County\tH1\n53179\t55059\tTrevor\tWI\tKenosha County\tH1\n53142\t55059\tKenosha\tWI\tKenosha County\tH1\n53181\t55059\tTwin lakes\tWI\tKenosha County\tH1\n53170\t55059\tSilver lake\tWI\tKenosha County\tH1\n53102\t55059\tBenet lake\tWI\tKenosha County\tH1\n53104\t55059\tBristol\tWI\tKenosha County\tH1\n53171\t55059\tSomers\tWI\tKenosha County\tH1\n53141\t55059\tKenosha\tWI\tKenosha County\tH1\n53177\t55059\tSturtevant\tWI\tKenosha County\tH1\n53101\t55059\tBassett\tWI\tKenosha County\tH1\n53194\t55059\tWoodworth\tWI\tKenosha County\tH1\n53152\t55059\tNew munster\tWI\tKenosha County\tH1\n53158\t55059\tPleasant prairie\tWI\tKenosha County\tH1\n53139\t55059\tKansasville\tWI\tKenosha County\tH1\n53143\t55059\tKenosha\tWI\tKenosha County\tH1\n53192\t55059\tWilmot\tWI\tKenosha County\tH1\n54205\t55061\tCasco\tWI\tKewaunee County\tH1\n54216\t55061\tKewaunee\tWI\tKewaunee County\tH1\n54213\t55061\tForestville\tWI\tKewaunee County\tH1\n54217\t55061\tLuxemburg\tWI\tKewaunee County\tH1\n54208\t55061\tDenmark\tWI\tKewaunee County\tH1\n54201\t55061\tAlgoma\tWI\tKewaunee County\tH1\n54667\t55063\tWestby\tWI\tLa Crosse County\tH1\n54603\t55063\tLa crosse\tWI\tLa Crosse County\tH1\n54669\t55063\tWest salem\tWI\tLa Crosse County\tH1\n54656\t55063\tSparta\tWI\tLa Crosse County\tH1\n54653\t55063\tRockland\tWI\tLa Crosse County\tH1\n54623\t55063\tCoon valley\tWI\tLa Crosse County\tH1\n54658\t55063\tStoddard\tWI\tLa Crosse County\tH1\n54642\t55063\tMelrose\tWI\tLa Crosse County\tH1\n54602\t55063\tLa crosse\tWI\tLa Crosse County\tH1\n54619\t55063\tCashton\tWI\tLa Crosse County\tH1\n54644\t55063\tMindoro\tWI\tLa Crosse County\tH1\n54601\t55063\tLa crosse\tWI\tLa Crosse County\tH1\n54650\t55063\tOnalaska\tWI\tLa Crosse County\tH1\n54636\t55063\tHolmen\tWI\tLa Crosse County\tH1\n54614\t55063\tBangor\tWI\tLa Crosse County\tH1\n53516\t55065\tBlanchardville\tWI\tLafayette County\tH1\n53522\t55065\tBrowntown\tWI\tLafayette County\tH1\n53807\t55065\tCuba city\tWI\tLafayette County\tH1\n53803\t55065\tBenton\tWI\tLafayette County\tH1\n53599\t55065\tWoodford\tWI\tLafayette County\tH1\n53530\t55065\tDarlington\tWI\tLafayette County\tH1\n53565\t55065\tMineral point\tWI\tLafayette County\tH1\n53586\t55065\tShullsburg\tWI\tLafayette County\tH1\n53818\t55065\tPlatteville\tWI\tLafayette County\tH1\n53811\t55065\tHazel green\tWI\tLafayette County\tH1\n53587\t55065\tSouth wayne\tWI\tLafayette County\tH1\n53504\t55065\tArgyle\tWI\tLafayette County\tH1\n53510\t55065\tBelmont\tWI\tLafayette County\tH1\n53541\t55065\tGratiot\tWI\tLafayette County\tH1\n54430\t55067\tElton\tWI\tLanglade County\tH1\n54465\t55067\tPickerel\tWI\tLanglade County\tH1\n54418\t55067\tBryant\tWI\tLanglade County\tH1\n54491\t55067\tWhite lake\tWI\tLanglade County\tH1\n54452\t55067\tMerrill\tWI\tLanglade County\tH1\n54424\t55067\tDeerbrook\tWI\tLanglade County\tH1\n54428\t55067\tElcho\tWI\tLanglade County\tH1\n54408\t55067\tAniwa\tWI\tLanglade County\tH1\n54462\t55067\tPearson\tWI\tLanglade County\tH1\n54409\t55067\tAntigo\tWI\tLanglade County\tH1\n54463\t55067\tPelican lake\tWI\tLanglade County\tH1\n54435\t55067\tGleason\tWI\tLanglade County\tH1\n54464\t55067\tPhlox\tWI\tLanglade County\tH1\n54414\t55067\tBirnamwood\tWI\tLanglade County\tH1\n54485\t55067\tSummit lake\tWI\tLanglade County\tH1\n54564\t55069\tTripoli\tWI\tLincoln County\tH1\n54452\t55069\tMerrill\tWI\tLincoln County\tH1\n54501\t55069\tRhinelander\tWI\tLincoln County\tH1\n54442\t55069\tIrma\tWI\tLincoln County\tH1\n54435\t55069\tGleason\tWI\tLincoln County\tH1\n54487\t55069\tTomahawk\tWI\tLincoln County\tH1\n54532\t55069\tHeafford junction\tWI\tLincoln County\tH1\n54126\t55071\tGreenleaf\tWI\tManitowoc County\tH1\n54220\t55071\tManitowoc\tWI\tManitowoc County\tH1\n54228\t55071\tMishicot\tWI\tManitowoc County\tH1\n54110\t55071\tBrillion\tWI\tManitowoc County\tH1\n54245\t55071\tValders\tWI\tManitowoc County\tH1\n53014\t55071\tChilton\tWI\tManitowoc County\tH1\n53015\t55071\tCleveland\tWI\tManitowoc County\tH1\n54215\t55071\tKellnersville\tWI\tManitowoc County\tH1\n54240\t55071\tTisch mills\tWI\tManitowoc County\tH1\n53042\t55071\tKiel\tWI\tManitowoc County\tH1\n54216\t55071\tKewaunee\tWI\tManitowoc County\tH1\n53063\t55071\tNewton\tWI\tManitowoc County\tH1\n54207\t55071\tCollins\tWI\tManitowoc County\tH1\n54241\t55071\tTwo rivers\tWI\tManitowoc County\tH1\n54232\t55071\tSaint nazianz\tWI\tManitowoc County\tH1\n54230\t55071\tReedsville\tWI\tManitowoc County\tH1\n53020\t55071\tElkhart lake\tWI\tManitowoc County\tH1\n54227\t55071\tMaribel\tWI\tManitowoc County\tH1\n54214\t55071\tFrancis creek\tWI\tManitowoc County\tH1\n54208\t55071\tDenmark\tWI\tManitowoc County\tH1\n54247\t55071\tWhitelaw\tWI\tManitowoc County\tH1\n53061\t55071\tNew holstein\tWI\tManitowoc County\tH1\n54474\t55073\tRothschild\tWI\tMarathon County\tH1\n54455\t55073\tMosinee\tWI\tMarathon County\tH1\n54412\t55073\tAuburndale\tWI\tMarathon County\tH1\n54451\t55073\tMedford\tWI\tMarathon County\tH1\n54473\t55073\tRosholt\tWI\tMarathon County\tH1\n54425\t55073\tDorchester\tWI\tMarathon County\tH1\n54423\t55073\tCuster\tWI\tMarathon County\tH1\n54417\t55073\tBrokaw\tWI\tMarathon County\tH1\n54452\t55073\tMerrill\tWI\tMarathon County\tH1\n54403\t55073\tWausau\tWI\tMarathon County\tH1\n54448\t55073\tMarathon\tWI\tMarathon County\tH1\n54440\t55073\tHatley\tWI\tMarathon County\tH1\n54479\t55073\tSpencer\tWI\tMarathon County\tH1\n54408\t55073\tAniwa\tWI\tMarathon County\tH1\n54427\t55073\tEland\tWI\tMarathon County\tH1\n54443\t55073\tJunction city\tWI\tMarathon County\tH1\n54411\t55073\tAthens\tWI\tMarathon County\tH1\n54488\t55073\tUnity\tWI\tMarathon County\tH1\n54401\t55073\tWausau\tWI\tMarathon County\tH1\n54409\t55073\tAntigo\tWI\tMarathon County\tH1\n54480\t55073\tStetsonville\tWI\tMarathon County\tH1\n54476\t55073\tSchofield\tWI\tMarathon County\tH1\n54471\t55073\tRingle\tWI\tMarathon County\tH1\n54449\t55073\tMarshfield\tWI\tMarathon County\tH1\n54421\t55073\tColby\tWI\tMarathon County\tH1\n54426\t55073\tEdgar\tWI\tMarathon County\tH1\n54402\t55073\tWausau\tWI\tMarathon County\tH1\n54429\t55073\tElderon\tWI\tMarathon County\tH1\n54484\t55073\tStratford\tWI\tMarathon County\tH1\n54414\t55073\tBirnamwood\tWI\tMarathon County\tH1\n54499\t55073\tWittenberg\tWI\tMarathon County\tH1\n54405\t55073\tAbbotsford\tWI\tMarathon County\tH1\n54157\t55075\tPeshtigo\tWI\tMarinette County\tH1\n54161\t55075\tPound\tWI\tMarinette County\tH1\n54156\t55075
